vi "Test_SerialPort.vi"() -> ()   [LabVIEW 2023, in "HAPS.lvlib"]
uses:
  HAPS.lvlib
  <vilib>/Instr/_visa.llb/VISA Configure Serial Port (Instr).vi
panel:
  out "Time(ms)":dbl
  out "Time(sec)":dbl
  out "bytes read 2":u32
  out "Response 2":string
  in  "Command":string="*IDN?\n"
  in  "Serial Settings":T1={"baud rate"=921600, "data bits"=8, "parity"=enum."None", "stop bits"=10, "flow control"=0} {"flow control" items=["None"=0, "XON/XOFF"=1, "RTS/CTS"=2, "DTR/DSR"=4]; "stop bits" items=["1.0"=10, "1.5"=15, "2.0"=20]; "data bits" min=5 max=8 step=1; "baud rate" items=["75"=75, "110"=110, "134"=134, "150"=150, "300"=300, "600"=600, "1200"=1200, "1800"=1800, "2400"=2400, "4800"=4800, "7200"=7200, "9600"=9600, "14400"=14400, "19200"=19200, "28800"=28800, "38400"=38400, "56000"=56000, "57600"=57600, "115200"=115200, "128000"=128000, "230400"=230400, "921600"=921600]}
  in  "delay before read (ms)":u32=5
  in  "VISA resource name":refnum<visa-resource-name>="COM1"
  out "bytes read":u32
  out "Response":string
  # "ch_ctrl_all\\s0,0,0,0\\r\\n"
  # "set_pd_range\\s0,0,0,9\\r\\n"
  # "get_bfic_temp\\s0,0,0\\r\\n"
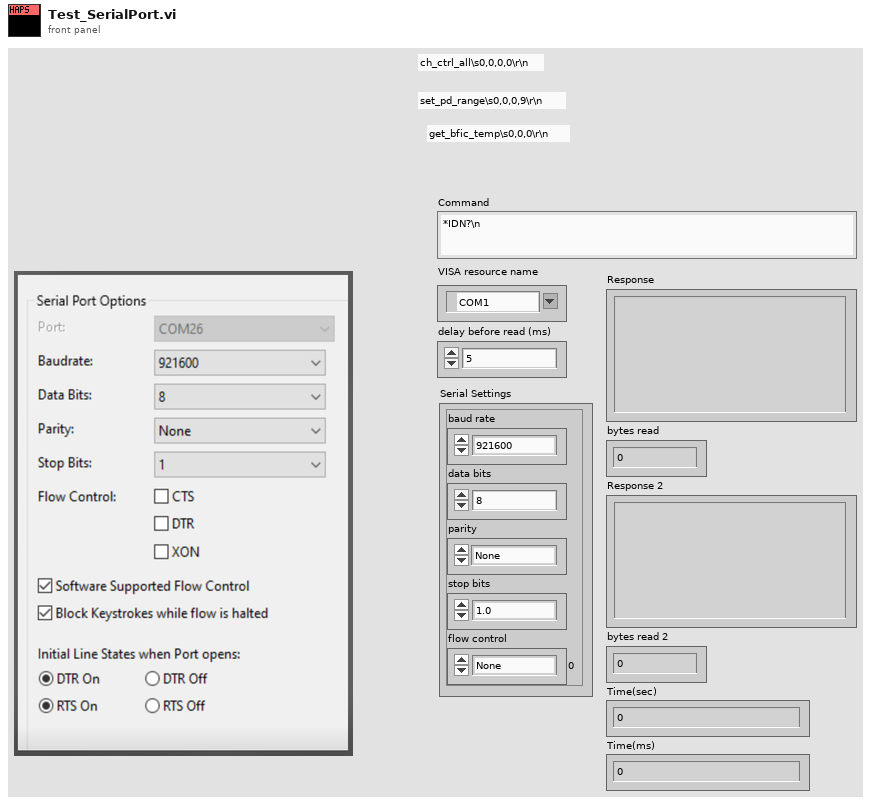
[diagram p1: front panel]
types:
  T1 = cluster{"baud rate":u32, "data bits":u16, "parity":enum16{"None", "Odd", "Even", "Mark", "Space"}, "stop bits":u16, "flow control":u16}
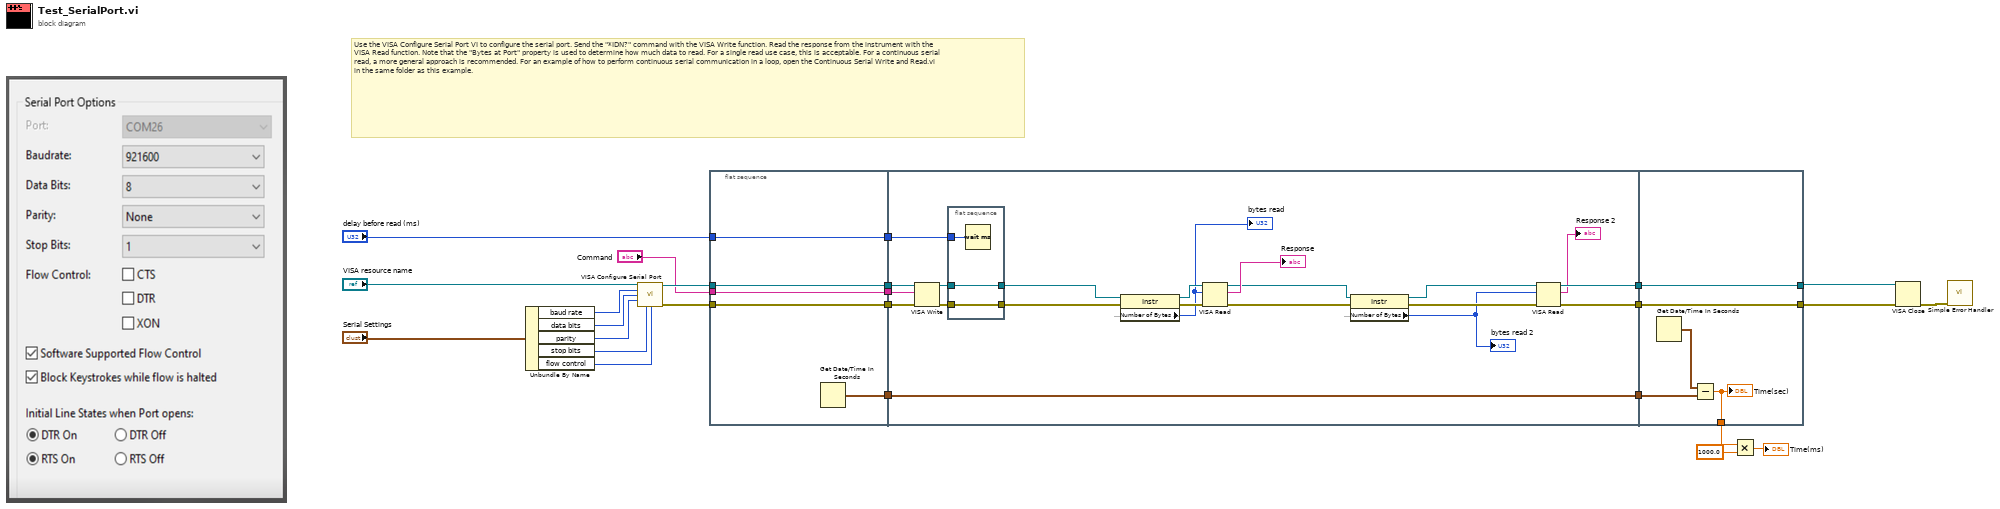
[diagram p0: block diagram]
diagram:
  # "Use the VISA Configure Serial Port VI to configure the serial port. Send the \"*IDN?\" command with the VISA Write function. Read the response from the instrument with the VISA Read function. Note that the \"Bytes at Port\" property is used to determine how much data to read. For a single read use case, this is acceptable. For a continuous serial read, a more general approach is recommended. For an example of how to perform continuous serial communication in a loop, open the Continuous Serial Write and Read.vi in the same folder as this example."
  n1 = Unbundle By Name("Serial Settings") -> ("baud rate"=w18:u32, "data bits"=w17:u16, "parity"=w16:enum16{"None", "Odd", "Even", "Mark", "Space"}, "stop bits"=w15:u16, "flow control"=w14:u16)
  n2 = call-poly "VISA Configure Serial Port"("VISA resource name"="VISA resource name", "baud rate (9600)"=w18, "data bits (8)"=w17, "parity (0:none)"=w16, "stop bits (10: 1 bit)"=w15, "flow control (0:none)"=w14) -> ("VISA resource name out"=w23:refnum<visa-resource-name>, "error out"=w24:errorcluster)  [unwired: 3 in, 5 out]
  n3 = flat-sequence {
    tunnel: "Command" -> [w27]
    tunnel: "delay before read (ms)" -> [w28]
    tunnel: w23 -> [w29]
    tunnel: w24 -> [w30]
    tunnel: [w30] -> w11
    tunnel: [w29] -> w10
    tunnel: [w28] -> w9
    tunnel: [w27] -> w8
    tunnel: [w26] -> w5
    tunnel: w11 -> [w51]
    tunnel: w10 -> [w50]
    tunnel: w9 -> [w47]
    tunnel: w8 -> [w46]
    tunnel: [w39] -> w7
    tunnel: [w38] -> w6
    tunnel: w5 -> [w31]
    tunnel: [w31] -> w4
    tunnel: [w58] -> w12
    tunnel: [w59] -> w13
    tunnel: w7 -> [w59]
    tunnel: w6 -> [w58]
    tunnel: w4 -> [w57]
    tunnel: [w55] -> w3
    frame #0 {
      n4 = Get Date/Time In Seconds() -> (seconds since 1Jan1904=w26:timestamp)
    }
    frame #1 {
      n5 = VISA Write(VISA resource name=w50, write buffer=w46, error in (no error)=w51) -> (VISA resource name out=w48:refnum<visa-resource-name>, error out=w49:errorcluster)  [unwired: 1 out]
      n6 = flat-sequence {
        tunnel: w49 -> [w53]
        tunnel: [w53] -> w42
        tunnel: w48 -> [w52]
        tunnel: [w52] -> w41
        tunnel: w47 -> [w54]
        frame #0 {
          n7 = Wait (ms)(milliseconds to wait=w54) -> ()  [unwired: 1 out]
        }
      }
      n8 = property class="Instr"(reference=w41, error in=w42) -> (reference out=w45:refnum<visa-resource-name>, error out=w44:errorcluster, "Serial Settings:Number of Bytes at Serial Port"=w40:u32)
      "bytes read" <- w40
      n9 = VISA Read(VISA resource name=w45, byte count=w40, error in (no error)=w44) -> (VISA resource name out=w37:refnum<visa-resource-name>, read buffer=→"Response":string, error out=w36:errorcluster)  [unwired: 1 out]
      n10 = property class="Instr"(reference=w37, error in=w36) -> (reference out=w34:refnum<visa-resource-name>, error out=w35:errorcluster, "Serial Settings:Number of Bytes at Serial Port"=w32:u32)
      "bytes read 2" <- w32
      n11 = VISA Read(VISA resource name=w34, byte count=w32, error in (no error)=w35) -> (VISA resource name out=w38:refnum<visa-resource-name>, read buffer=→"Response 2":string, error out=w39:errorcluster)  [unwired: 1 out]
    }
    frame #2 {
      n12 = Get Date/Time In Seconds() -> (seconds since 1Jan1904=w56:timestamp)
      n13 = Subtract(x=w56, y=w57) -> (x-y=w55:dbl)
      "Time(sec)" <- w55
    }
  }
  n14 = Multiply(x=w3, y=1000.0) -> (x*y=→"Time(ms)":dbl)
  n15 = VISA Close(VISA resource name=w12, error in (no error)=w13) -> (error out=w22:errorcluster)
  n16 = call <vilib>:"Simple Error Handler.vi"("error in (no error)"=w22) -> ()  [unwired: 1 in, 8 out]
